vi "Initialize.vi"(8 "error in (no error)":errorcluster, 11 "physical channels":tag="Dev1/ai1") -> (0 "error out":errorcluster, 3 "task out":refnum<k21>)   [LabVIEW 2018, in "Pressure Actor.lvlib" / "Pressure.lvclass"]
uses:
  Pressure.lvclass
  <vilib>/DAQmx/create/channels.llb/DAQmx Create Channel (AI-Voltage-Basic).vi
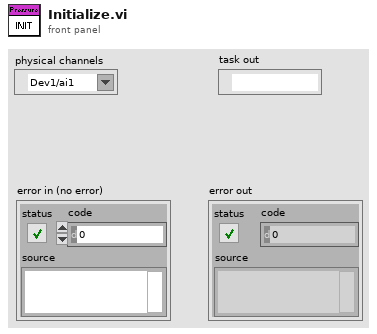
[diagram p1: front panel]
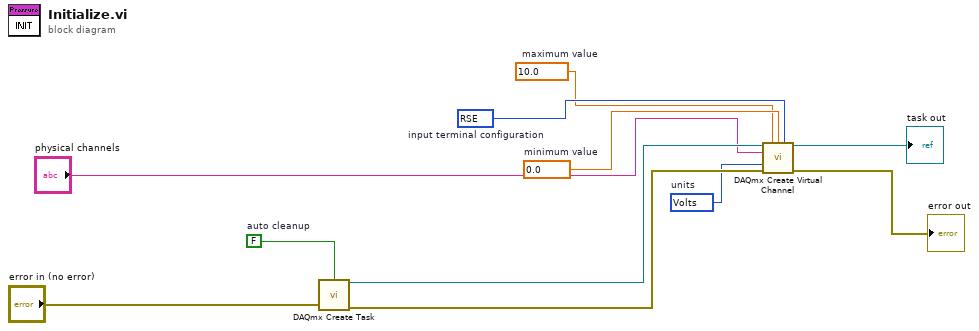
[diagram p0: block diagram]
diagram:
  w8 = 10083 items=["default"=-1, "RSE"=10083, "NRSE"=10078, "Differential"=10106, "Pseudodifferential"=12529]  # input terminal configuration
  w6 = 10348 items=["Volts"=10348, "From Custom Scale"=10065]  # units
  w7 = 0.0  # minimum value
  w4 = 10.0  # maximum value
  w10 = FALSE  # auto cleanup
  n1 = call <vilib>:"DAQmx Create Task.vi"("auto cleanup"=w10, "error in"="error in (no error)") -> ("task out"=w11:refnum<k21>, "error out"=w9:errorcluster)  [unwired: 12 in]
  n2 = call-poly <vilib>:"DAQmx Create Virtual Channel.vi"("task in"=w11, "maximum value"=w4, "minimum value"=w7, "input terminal configuration"=w8, "physical channels"="physical channels", "units"=w6, "error in"=w9) -> ("task out"=→"task out":refnum<k21>, "error out"=→"error out":errorcluster)  [unwired: 7 in]
